vi "SetExternalInterfaces.vi"(8 "ErrorIn":errorcluster, 10 "ExternalInterfaces":T1[](array[typedef]), 11 "ReferenceIn":refnum<class "UserManager.lvclass">) -> (0 "ErrorOut":errorcluster, 3 "ReferenceOut":refnum<class "UserManager.lvclass">)   [LabVIEW 2021, in "UserMananger.lvlib" / "UserManager.lvclass"]
uses:
  UserManager.lvclass
  Library_TAF_Support/ClusterArrayConversion/BundledArray.ctl
  0a6ec689-4898-488c-8e07-ed5616c8d135.vi
  0a6ec689-4898-488c-8e07-ed5616c8d135.vi/e733eca7-9823-4359-8665-3b184f9a7377.vi
  0a6ec689-4898-488c-8e07-ed5616c8d135.vi/185eb5ab-e8f7-4395-854b-f566a9b9020c.vi
  <vilib>/Utility/Data Type/Get Cluster Information.vi
  <vilib>/Utility/Data Type/Get Type Information.vi
  <userlib>/_OpenG.lib/lvdata/lvdata.llb/Array of VData to VCluster__ogtk.vi
  <vilib>/Utility/LVClass/Get LV Class Name.vi
  UserManager.lvclass/UserManager.ctl
  Library_TAF_Support/ClusterArrayConversion/ClusterArrayConversion.lvlib
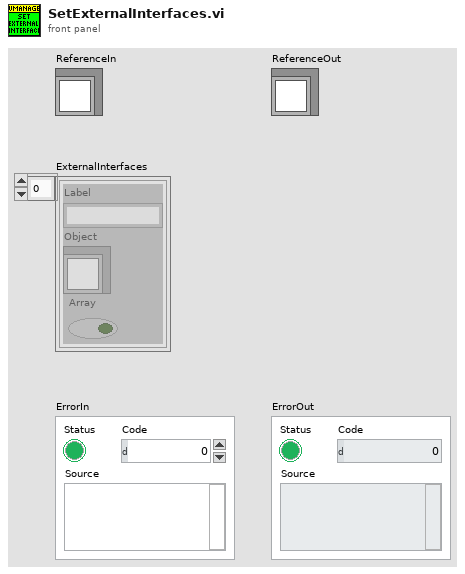
[diagram p1: front panel]
types:
  T1 = typedef "ClusterArrayConversion.lvlib/BundledArray.ctl" = cluster{"Label":string, "Object":refnum<class>, "Array":bool}
  T2 = typedef "UserMananger.lvlib/UserManager.lvclass/ObjectAttributes.ctl" = cluster{"Interfaces":cluster{"ActivationUpdated":refnum<class "IAuthorizationUpdated.lvclass">}, "Locals":cluster{"MainGUIActive":refnum<queue>, "Evaluations":cluster{"Label":string, "Value":string}[]}, "Persistent":cluster{"Dummy":bool}}
  T3 = cluster{"ActivationUpdated":refnum<class "IAuthorizationUpdated.lvclass">}
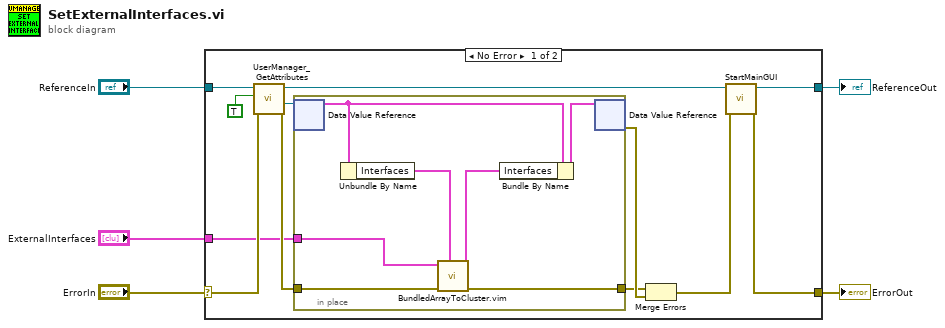
[diagram p0: block diagram]
diagram:
  n1 = case shown="No Error" "ErrorIn" {
    selector: "ErrorIn" -> [w17 w26]
    tunnel: [w12 w26] -> w4
    tunnel: [w6 w25] -> w2
    tunnel: "ReferenceIn" -> [w11 w25]
    tunnel: "ExternalInterfaces" -> [w7 _]
    frame No Error {
      n2 = call "UserManager_GetAttributes.vi"("ErrorIn"=w17, "OnlyGetDvrReference(False)"=TRUE, "ReferenceIn"=w11) -> ("ErrorOut"=w14:errorcluster, "DataRef"=w8:refnum<data-value>, "ReferenceOut"=w10:refnum<class "UserManager.lvclass">)  [unwired: 5 in, 1 out]
      n3 = in-place {
        in-place-border: [w24] -> w15
        in-place-border: w14 -> [w23]
        in-place-border: w7 -> [w18]
        n4 = in-place-dvr #1(w8) -> (w21:T2)  [unwired: 1 out]
        n5 = Unbundle By Name(w21) -> ("Interfaces"=w20:T3)
        n6 = call "BundledArrayToCluster.vim"("Type"=w20, "ErrorIn"=w23, "BundeledLabels"=w18) -> ("ErrorOut"=w24:errorcluster, "DataOut"=w19:T3)  [unwired: 7 in]
        n7 = Bundle By Name(cluster=w21, "Interfaces"=w19) -> (w22:T2)
        n8 = in-place-dvr #1(w22) -> (w16:errorcluster)  [unwired: 1 out]
      }
      n9 = Merge Errors(w15, w16) -> (w13:errorcluster)
      n10 = call "StartMainGUI.vi"("ErrorIn"=w13, "ReferenceIn"=w10) -> ("ErrorOut"=w12:errorcluster, "ReferenceOut"=w6:refnum<class "UserManager.lvclass">)  [unwired: 6 in, 2 out]
    }
    frame Error {
    }
  }
  "ErrorOut" <- w4
  "ReferenceOut" <- w2
